vi "Prompt.vi"() -> (2 "Cluster":T1)   [LabVIEW 2013, in "Data Logger.lvlib" / "Data Logger.lvclass"]
uses:
  Data Logger.lvclass
panel:
  in  "Done Button":bool
  in  "Comment":string
  in  "Serial":string
  in  "Model":string
  in  "Project Number":string
  in  "Manufacturer":string
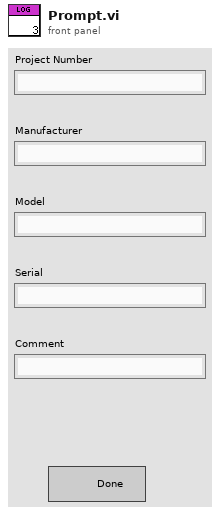
[diagram p1: front panel]
types:
  T1 = cluster{"Project Number":string, "Manufacturer":string, "Model":string, "Serial":string, "Comment":string}
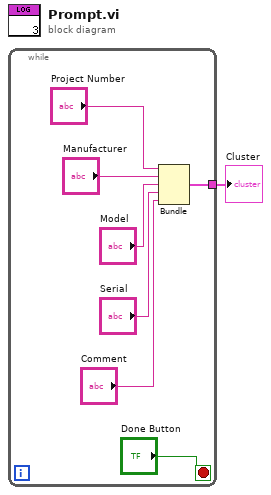
[diagram p0: block diagram]
diagram:
  n1 = while {
    tunnel: [w5] -> w1
    stop <- "Done Button" stop-if-true
    n2 = Bundle("Project Number"="Project Number", "Manufacturer"="Manufacturer", "Model"="Model", "Serial"="Serial", "Comment"="Comment") -> (w5:T1)  [unwired: 1 in]
  }
  "Cluster" <- w1
